vi "LHF.DB.Mongo.Util.FindRegex.vi"(6 "regex":string, 8 "error in (no error)":errorcluster, 9 "name":string, 10 "Collection":string, 11 "LHF.DB.Mongo in":refnum<class "LHF.DB.Mongo.lvclass">) -> (0 "error out":errorcluster, 2 "Documents":string[](array[string]), 3 "LHF.DB.Mongo out":refnum<class "LHF.DB.Mongo.lvclass">, 5 "ObjectIDs":string[](array[string]))   [LabVIEW 2013, in "LHF.DB.Mongo.lvclass"]
uses:
  LHF.DB.Mongo.lvclass
  C:/Users/schim/Desktop/Projetos/LabVIEW-MongoDB/src/Driver/MongoDB.Bson.dll
  Driver/MongoDB.Bson.dll
  C:/Users/schim/Desktop/Projetos/LabVIEW-MongoDB/src/Driver/MongoDB.Driver.dll
  Driver/MongoDB.Driver.dll
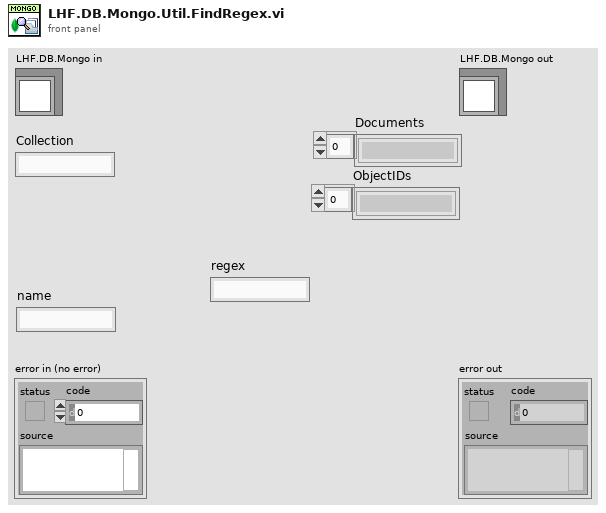
[diagram p1: front panel]
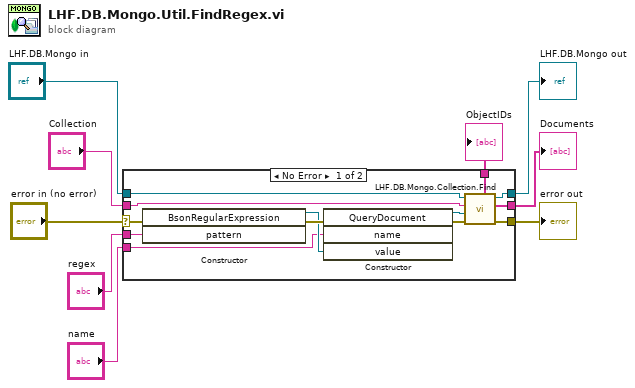
[diagram p0: block diagram]
diagram:
  n1 = case shown="No Error" "error in (no error)" {
    selector: "error in (no error)" -> [w21 w24]
    tunnel: [w14 w24] -> w8
    tunnel: [w16 w23] -> w6
    tunnel: "LHF.DB.Mongo in" -> [w17 w23]
    tunnel: "Collection" -> [w11 _]
    tunnel: "name" -> [w18 _]
    tunnel: [w15 _] -> w3
    tunnel: "regex" -> [w20 _]
    tunnel: [w10 _] -> w1
    frame No Error {
      n2 = constructor class="BsonRegularExpression"(error in=w21, "pattern"=w20) -> (reference out=w19:refnum<k24>, error out=w22:errorcluster)  [unwired: 2 in, 2 out]
      n3 = constructor class="QueryDocument"(error in=w22, "name"=w18, "value"=w19) -> (reference out=w12:refnum<k24>, error out=w13:errorcluster)  [unwired: 2 in, 3 out]
      n4 = call "LHF.DB.Mongo.Collection.Find.vi"("error in (no error)"=w13, "query"=w12, "Collection"=w11, "LHF.DB.Mongo in"=w17) -> ("error out"=w14:errorcluster, "Documents"=w15:string[], "LHF.DB.Mongo out"=w16:refnum<class "LHF.DB.Mongo.lvclass">, "ObjectIDs"=w10:string[])  [unwired: 4 in]
    }
    frame Error {
    }
  }
  "error out" <- w8
  "LHF.DB.Mongo out" <- w6
  "Documents" <- w3
  "ObjectIDs" <- w1
